vi "CalculateDaysSince.vi"() -> ()   [LabVIEW 2018]
panel:
  in  "Date":T1={"day"=1, "month"=enum."May", "year"=2019}
  out "days since date":i32
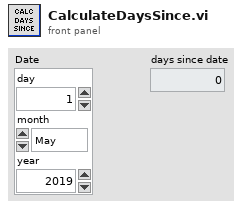
[diagram p1: front panel]
types:
  T1 = cluster{"day":i32, "month":enum16{"Jan", "Feb", "Mar", "Apr", "May", "Jun", "Jul", "Aug", "Sept", "Oct", "Nov", "Dec"}, "year":i32}
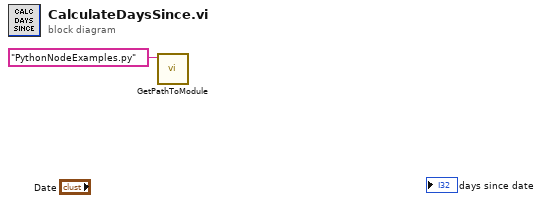
[diagram p0: block diagram]
diagram:
  n1 = call "GetPathToModule.vi"("module name"="PythonNodeExamples.py") -> ()  [unwired: 10 in, 1 out]
